vi "Destroy Class.vi"(8 "error in (no error)":errorcluster, 11 "Stage Data Class":refnum<data-value>) -> (0 "error out":errorcluster)   [LabVIEW 2022 SP3, in "XY Stage Data Class.lvclass"]
uses:
  XY Stage Data Class.lvclass
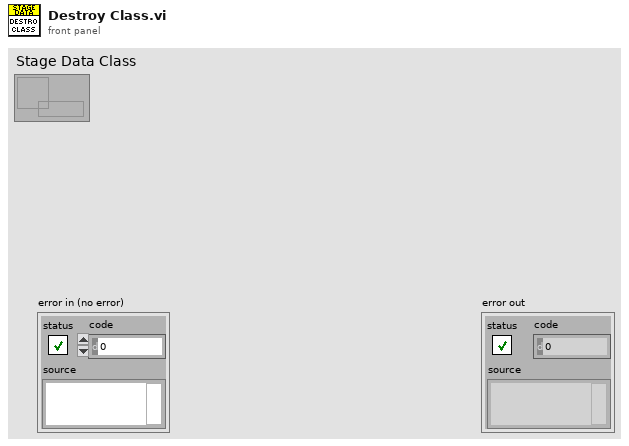
[diagram p1: front panel]
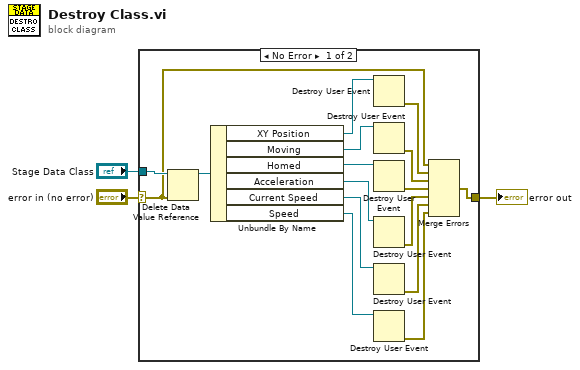
[diagram p0: block diagram]
diagram:
  n1 = case shown="No Error" "error in (no error)" {
    selector: "error in (no error)" -> [w18 w20]
    tunnel: [w10 w20] -> w2
    tunnel: "Stage Data Class" -> [w19 _]
    frame No Error {
      n2 = Delete Data Value Reference(data value reference=w19, error in=w18) -> (data value=w17:refnum<class "XY Stage Data Class.lvclass">)  [unwired: 1 out]
      n3 = Unbundle By Name(w17) -> ("XY Position"=w16:refnum<user-event>, "Moving"=w15:refnum<user-event>, "Homed"=w14:refnum<user-event>, "Acceleration"=w13:refnum<user-event>, "Current Speed"=w12:refnum<user-event>, "Speed"=w11:refnum<user-event>)
      n4 = Destroy User Event(user event=w16) -> (error out=w9:errorcluster)  [unwired: 1 in]
      n5 = Destroy User Event(user event=w15) -> (error out=w8:errorcluster)  [unwired: 1 in]
      n6 = Destroy User Event(user event=w14) -> (error out=w7:errorcluster)  [unwired: 1 in]
      n7 = Destroy User Event(user event=w13) -> (error out=w6:errorcluster)  [unwired: 1 in]
      n8 = Destroy User Event(user event=w12) -> (error out=w5:errorcluster)  [unwired: 1 in]
      n9 = Destroy User Event(user event=w11) -> (error out=w4:errorcluster)  [unwired: 1 in]
      n10 = Merge Errors(w18, w9, w8, w7, w6, w5, w4) -> (w10:errorcluster)
    }
    frame Error {
    }
  }
  "error out" <- w2
